vi "H-Drive Actuation.vi"(10 "Button 5":bool, 11 "Button 4":bool) -> ()   [LabVIEW 2014]
uses:
  <vilib>/Rock Robotics/WPI/Solenoid/Deprecated/WPI_SolenoidSetBool.vi
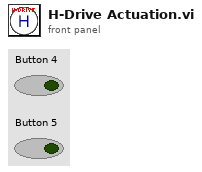
[diagram p1: front panel]
types:
  T1 = typedef "WPI_SolenoidDevRef.ctl" = cluster{"DevStatus":errorcluster, "Pneumatics Control Module":u8, "Forward Solenoid Channel":T2, "Reverse Solenoid Channel":T2}
  T2 = typedef "WPI_SolenoidChannel.ctl" = enum8{"Solenoid 0", "Solenoid 1", "Solenoid 2", "Solenoid 3", "Solenoid 4", "Solenoid 5", "Solenoid 6", "Solenoid 7", "Invalid"}
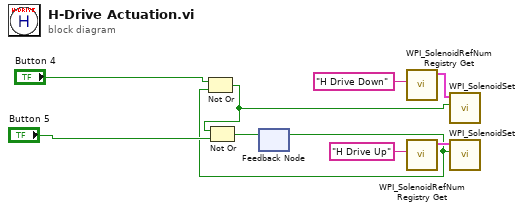
[diagram p0: block diagram]
diagram:
  n1 = feedback #1() -> (w1:bool)  [unwired: 1 in]
  n2 = Not Or(1:w1, 2:"Button 4") -> (0:w2:bool)
  n3 = Not Or(1:"Button 5", 2:w2) -> (0:w3:bool)
  n4 = feedback-in #1(w3) -> ()
  n5 = call <vilib>:"WPI_SolenoidRefNum Registry Get.vi"("refnum name"="H Drive Down") -> ("SolenoidDevRef"=w7:T1)  [unwired: 9 in, 1 out]
  n6 = call <vilib>:"WPI_SolenoidRefNum Registry Get.vi"("refnum name"="H Drive Up") -> ("SolenoidDevRef"=w8:T1)  [unwired: 9 in, 1 out]
  n7 = call-poly <vilib>:"WPI_SolenoidSet.vi"("Value"=w2, "SolenoidDevRef"=w7) -> ()  [unwired: 8 in, 2 out]
  n8 = call-poly <vilib>:"WPI_SolenoidSet.vi"("Value"=w1, "SolenoidDevRef"=w8) -> ()  [unwired: 8 in, 2 out]
